vi "eDIDS-24XX-FPGA1-EPTx.vi"() -> ()   [LabVIEW 2015, in "ECS-FPGA.lvlib"]
uses:
  ECS-FPGA.lvlib
  <vilib>/Powertrain Controls/Device Drivers/Engine Position Tracking/EPTx/RevA/FPGA/Controls/EPTxTooth.ctl
  <vilib>/Powertrain Controls/Device Drivers/Engine Position Tracking/EPTx/RevA/FPGA/Controls/EPTxControl.ctl
  <vilib>/Powertrain Controls/Device Drivers/Engine Position Tracking/EPTx/RevA/FPGA/Controls/EPTxConfig.ctl
  <vilib>/Powertrain Controls/Device Drivers/Engine Position Tracking/EPTx/RevA/FPGA/Controls/EPTxSupervisor.ctl
  <vilib>/Powertrain Controls/Device Drivers/Engine Position Tracking/EPTx/RevA/FPGA/Controls/EPTxAAPControl.ctl
  <vilib>/Platform/TimedLoop/XDataNode/timing_clust.ctl
  <vilib>/Platform/TimedLoop/XDataNode/nitl_modes.ctl
  <vilib>/Platform/TimedLoop/XDataNode/wakeup.ctl
  <vilib>/Powertrain Controls/Device Drivers/Engine Position Tracking/EPTx/RevA/FPGA/Controls/EPTxSignals.ctl
  <vilib>/rvi/Emulation/niFpgaGetClockAttributes.vi
  <vilib>/rvi/Emulation/niFpgaSctlEmulationGetInTimedLoop.vi
  <vilib>/rvi/Emulation/niFpgaEmulationReportErrorSimple.vi
  <vilib>/rvi/eio/common/nirviEmuTemplateMethod_errors.vi
  <vilib>/rvi/Emulation/niFpgaCriticalErrorInLSC.vi
  <vilib>/eio/EIONode/EIONode.xnode
  <vilib>/Platform/TimedLoop/XDataNode/XDataNode.xnode
  <vilib>/Platform/TimedLoop/XDataNode/XDNodeRunTimeDep.lvlib
  <vilib>/Powertrain Controls/Device Drivers/Engine Position Tracking/EPTx/RevA/FPGA/EPTx - RevA - FPGA.lvlib
panel:
  in  "EPTx.Aux4":u8
  in  "EPTx.Aux2":u8
  in  "DI-4.PlsGen_Config_Channel3":T1
  in  "DI-4.PlsGen_Config_Channel2":T1
  in  "DI-4.PlsGen_Config_Channel1":T1
  out "DI-4.Data":T2 caption="DIData"
  out "DI-4.ScopeData":T3 caption="DIScopeData"
  in  "DI-4.ScopeRead":bool caption="DIScopeRead"
  in  "DI-4.IPhaseInterface":T4(array[cluster]) caption="IPhaseInterface"
  in  "DI-4.Control":T5 caption="DIControl"
  in  "DI-3.PlsGen_Config_Channel3":T1
  in  "DI-3.PlsGen_Config_Channel2":T1
  in  "DI-3.PlsGen_Config_Channel1":T1
  out "DI-3.Data":T2 caption="DIData"
  out "DI-3.ScopeData":T3 caption="DIScopeData"
  in  "DI-3.ScopeRead":bool caption="DIScopeRead"
  in  "DI-3.IPhaseInterface":T4(array[cluster]) caption="IPhaseInterface"
  in  "DI-3.Control":T5 caption="DIControl"
  in  "DI-2.PlsGen_Config_Channel3":T1
  in  "DI-2.PlsGen_Config_Channel2":T1
  in  "DI-2.PlsGen_Config_Channel1":T1
  out "DI-2.Data":T2 caption="DIData"
  out "DI-2.ScopeData":T3 caption="DIScopeData"
  in  "DI-2.ScopeRead":bool caption="DIScopeRead"
  in  "DI-2.IPhaseInterface":T4(array[cluster]) caption="IPhaseInterface"
  in  "DI-2.Control":T5 caption="DIControl"
  in  "DI-1.Control":T5 caption="DIControl"
  in  "DI-1.IPhaseInterface":T4(array[cluster]) caption="IPhaseInterface"
  in  "DI-1.ScopeRead":bool caption="DIScopeRead"
  out "DI-1.ScopeData":T3 caption="DIScopeData"
  out "DI-1.Data":T2 caption="DIData"
  in  "DI-1.PlsGen_Config_Channel1":T1
  in  "DI-1.PlsGen_Config_Channel2":T1
  in  "DI-1.PlsGen_Config_Channel3":T1
  in  "EPTx.Aux1AngleCapture":T6
  in  "EPTx.Aux2AngleCapture":T6
  out "EPTx.Aux1EdgeCount":u8
  out "EPTx.Aux2EdgeCount":u8
  out "EPTx.Aux1CaptureCAD":fxp<+,18,11>
  out "EPTx.Aux2CaptureCAD":fxp<+,18,11>
  in  "EPTx.Aux3AngleCapture":T6
  in  "EPTx.Aux4AngleCapture":T6
  out "EPTx.Aux3EdgeCount":u8
  out "EPTx.Aux4EdgeCount":u8
  out "EPTx.Aux3CaptureCAD":fxp<+,18,11>
  out "EPTx.Aux4CaptureCAD":fxp<+,18,11>
  in  "EPTx.Aux3":u8
  in  "EPTx.Primary":u8
  in  "EPTx.Aux1":u8
  out "EPTxSupervisor":T7
  in  "EPTxConfig":T8
  in  "EPTxControl":T9
  out "EPTxTooth":T10
  out "9411-2.DigitalTriggers":u32
  out "9220-1/AI15":fxp<+/-,24,5>
  out "9220-1/AI14":fxp<+/-,24,5>
  out "9220-1/AI13":fxp<+/-,24,5>
  out "9220-1/AI12":fxp<+/-,24,5>
  out "9220-1/AI11":fxp<+/-,24,5>
  out "9220-1/AI10":fxp<+/-,24,5>
  out "9220-1/AI9":fxp<+/-,24,5>
  out "9220-1/AI8":fxp<+/-,24,5>
  out "9220-1/AI7":fxp<+/-,24,5>
  out "9220-1/AI6":fxp<+/-,24,5>
  out "9220-1/AI5":fxp<+/-,24,5>
  out "9220-1/AI4":fxp<+/-,24,5>
  out "9220-1/AI3":fxp<+/-,24,5>
  out "9220-1/AI2":fxp<+/-,24,5>
  out "9220-1/AI1":fxp<+/-,24,5>
  out "9220-1/AI0":fxp<+/-,24,5>
  out "9411-2.5.PPWData":T11
  out "9411-2.4.PPWData":T11
  out "9411-2.3.PPWData":T11
  out "9411-2.2.PPWData":T11
  out "9411-2.1.PPWData":T11
  out "9411-2.0.PPWData":T11
  out "9411-1.5.PPWData":T11
  out "9411-1.4.PPWData":T11
  out "9411-1.3.PPWData":T11
  out "9411-1.2.PPWData":T11
  out "9411-1.1.PPWData":T11
  out "9411-1.0.PPWData":T11
  out "9411-1.DigitalTriggers":u32
  in  "9411-2.0.Filt":u16
  in  "9411-2.1.Filt":u16
  in  "9411-2.2.Filt":u16
  in  "9411-2.3.Filt":u16
  in  "9411-2.4.Filt":u16
  in  "9411-2.5.Filt":u16
  in  "9411-2.Invert":u8
  in  "9411-1.0.Filt":u16
  in  "9411-1.1.Filt":u16
  in  "9411-1.2.Filt":u16
  in  "9411-1.3.Filt":u16
  in  "9411-1.4.Filt":u16
  in  "9411-1.5.Filt":u16
  in  "9411-1.Invert":u8
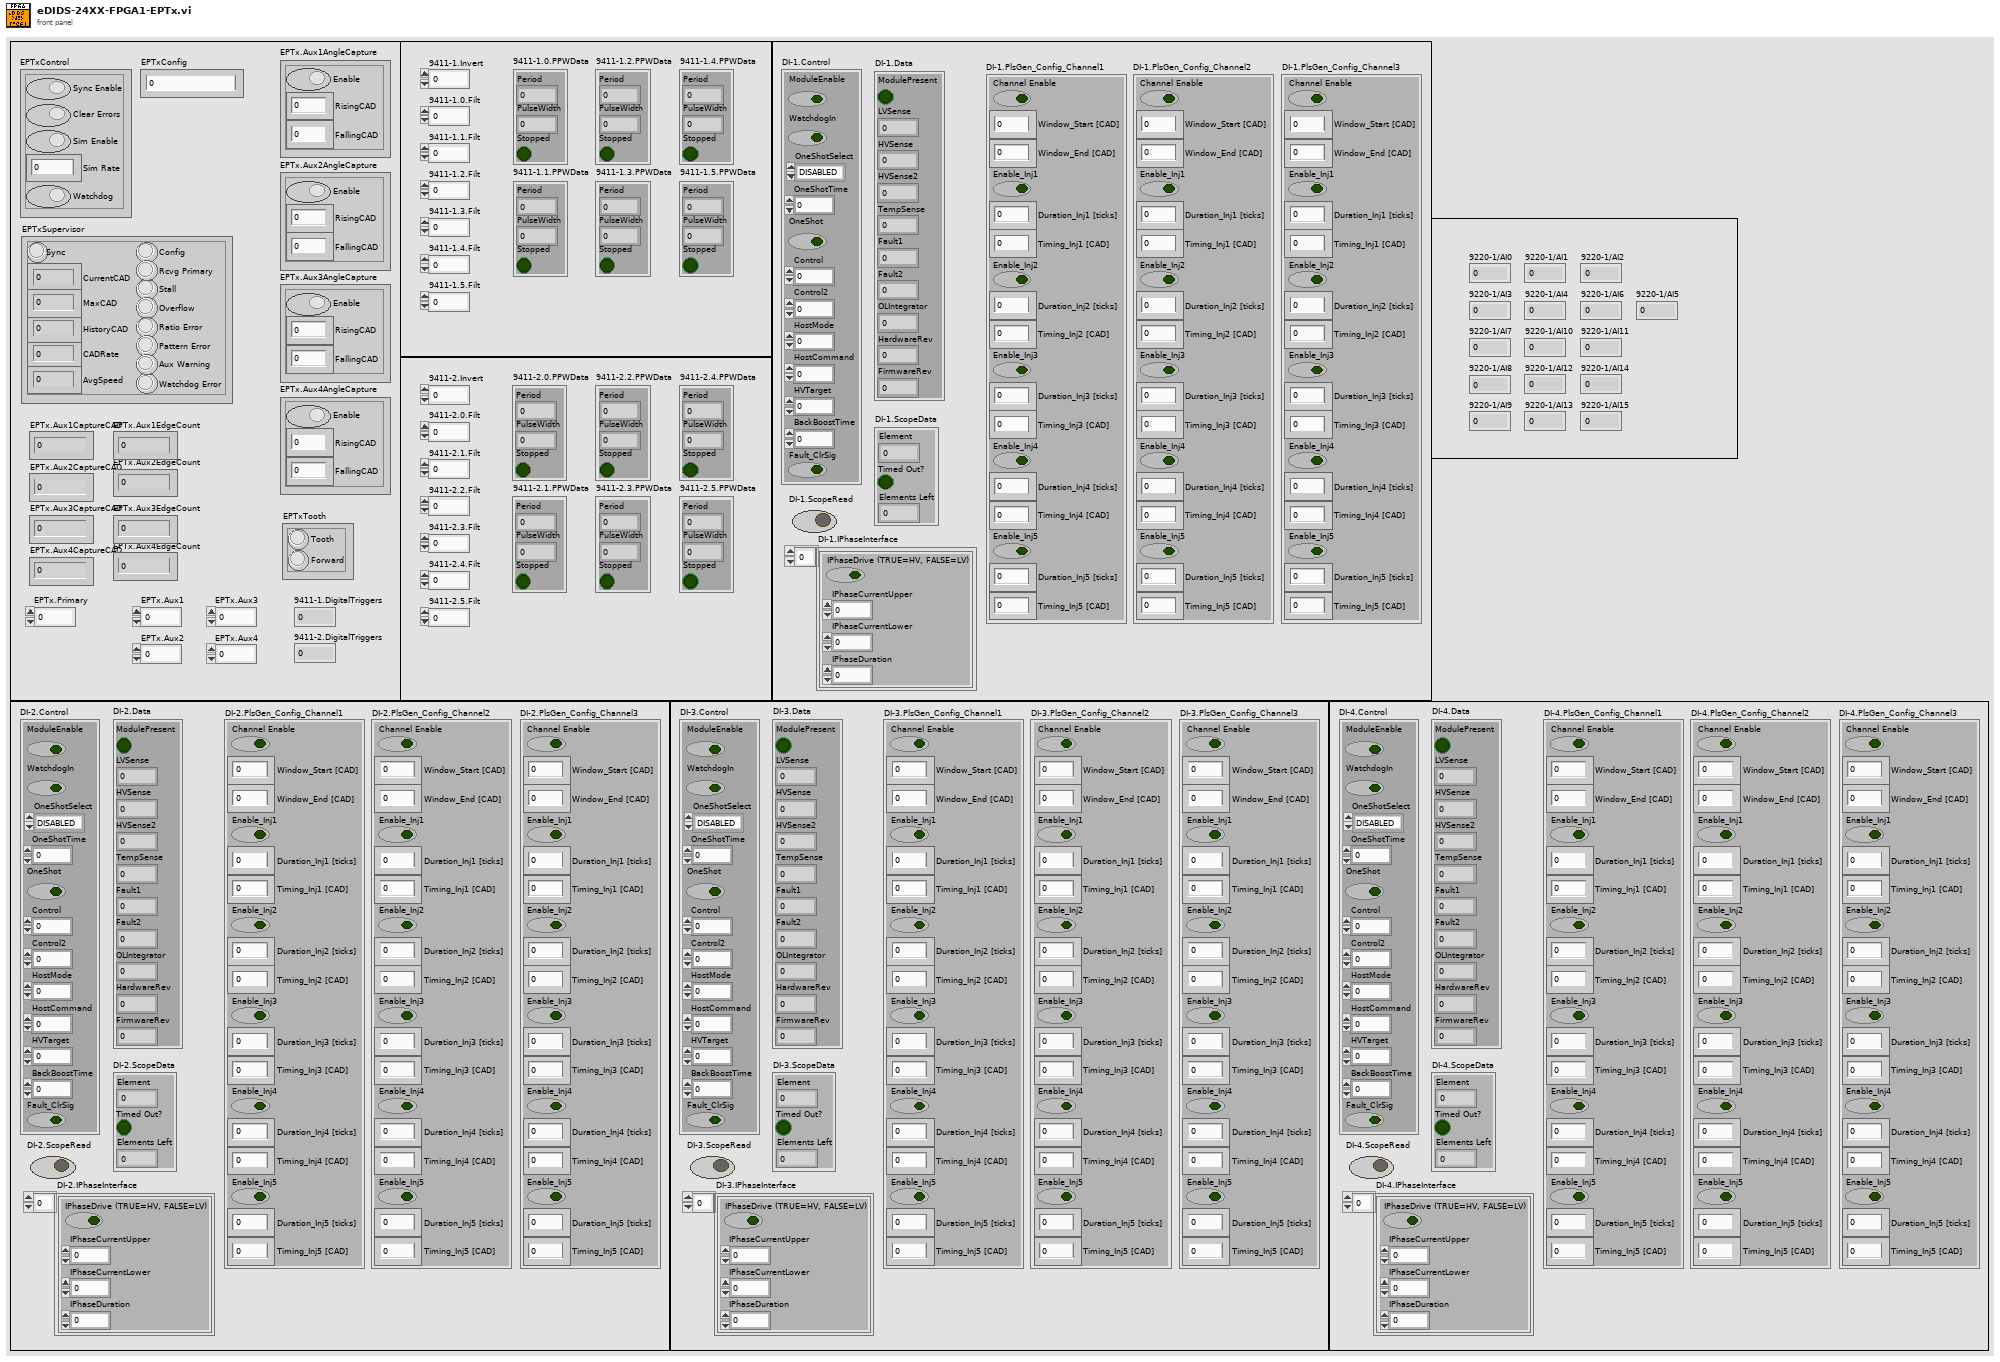
[diagram p1: front panel]
types:
  T1 = cluster{"Channel Enable":bool, "Window_Start [CAD]":fxp<+,18,11>, "Window_End [CAD]":fxp<+,18,11>, "Enable_Inj1":bool, "Duration_Inj1 [ticks]":u32, "Timing_Inj1 [CAD]":fxp<+,18,11>, "Enable_Inj2":bool, "Duration_Inj2 [ticks]":u32, "Timing_Inj2 [CAD]":fxp<+,18,11>, "Enable_Inj3":bool, "Duration_Inj3 [ticks]":u32, "Timing_Inj3 [CAD]":fxp<+,18,11>, "Enable_Inj4":bool, "Duration_Inj4 [ticks]":u32, "Timing_Inj4 [CAD]":fxp<+,18,11>, "Enable_Inj5":bool, "Duration_Inj5 [ticks]":u32, "Timing_Inj5 [CAD]":fxp<+,18,11>}
  T2 = cluster{"ModulePresent":bool, "LVSense":u8, "HVSense":u8, "HVSense2":u8, "TempSense":i8, "Fault1":u8, "Fault2":u8, "OLIntegrator":u32, "HardwareRev":u8, "FirmwareRev":u8}
  T3 = cluster{"Element":u32, "Timed Out?":bool, "Elements Left":u32}
  T4 = cluster{"IPhaseDrive (TRUE=HV, FALSE=LV)":bool, "IPhaseCurrentUpper":u16, "IPhaseCurrentLower":u16, "IPhaseDuration":u16}[]
  T5 = cluster{"ModuleEnable":bool, "WatchdogIn":bool, "OneShotSelect":enum8{"DISABLED", "CHAN 1", "CHAN 2", "CHAN 3"}, "OneShotTime":u32, "OneShot":bool, "Control":u8, "Control2":u8, "HostMode":u8, "HostCommand":u32, "HVTarget":u8, "BackBoostTime":u8, "Fault_ClrSig":bool}
  T6 = typedef "EPTx - RevA - FPGA.lvlib/EPTxAAPControl.ctl" = cluster{"Enable":bool, "RisingCAD":fxp<+,18,11>, "FallingCAD":fxp<+,18,11>}
  T7 = typedef "EPTx - RevA - FPGA.lvlib/EPTxSupervisor.ctl" = cluster{"Sync":bool, "CurrentCAD":fxp<+,18,11>, "MaxCAD":fxp<+,11,11>, "HistoryCAD":fxp<+,11,11>, "CADRate":fxp<+,22,8>, "AvgSpeed":fxp<+,17,15>, "Config":bool, "Rcvg Primary":bool, "Stall":bool, "Overflow":bool, "Ratio Error":bool, "Pattern Error":bool, "Aux Warning":bool, "Watchdog Error":bool}
  T8 = typedef "EPTx - RevA - FPGA.lvlib/EPTxConfig.ctl" = u64
  T9 = typedef "EPTx - RevA - FPGA.lvlib/EPTxControl.ctl" = cluster{"Sync Enable":bool, "Clear Errors":bool, "Sim Enable":bool, "Sim Rate":fxp<+,24,6>, "Watchdog":bool}
  T10 = typedef "EPTx - RevA - FPGA.lvlib/EPTxTooth.ctl" = cluster{"Tooth":bool, "Forward":bool}
  T11 = cluster{"Period":u32, "PulseWidth":u32, "Stopped":bool}
  T12 = typedef "XDNodeRunTimeDep.lvlib/timing_clust.ctl" = cluster{"Expected End [f-1]":u64, "Actual End [f-1]":u64, "Finished Late? [f-1]":bool, "Expected End [i-1]":u64, "Actual End [i-1]":u64, "Finished Late? [i-1]":bool, "Expected Start [i]":u64, "Actual Start [i]":u64, "Expected Start [f]":u64, "Actual Start [f]":u64, "Source Name":string, "Structure Name":string, "Period":i64, "Deadline":i64, "Offset":i64, "Start":i64, "Priority":i32, "Timeout":i32, "Mode":T13, "Wakeup Reason":T14, "Error":errorcluster, "Source Type":string, "Secondary Source Type":string, "Global End Time":u64, "Global Start Time":u64, "Frame Duration":u64, "Iteration Duration":u64, "Assigned CPU":i32, "I/O Scan Engine Mode":u32}
  T13 = typedef "XDNodeRunTimeDep.lvlib/nitl_modes.ctl" = enum32{"No Change", "Process missed periods, maintain original phase", "Discard missed periods, maintain original phase", "Process missed periods, ignore original phase", "Discard missed periods, ignore original phase"}
  T14 = typedef "XDNodeRunTimeDep.lvlib/wakeup.ctl" = enum32{"Normal", "Aborted", "Asynchronous wakeup", "Timing source error", "Timed loop error", "Timeout"}
  T15 = typedef "EPTx - RevA - FPGA.lvlib/EPTxSignals.ctl" = cluster{"Primary":bool, "Aux 1":bool, "Aux 2":bool, "Aux 3":bool, "Aux 4":bool}
  T16 = cluster{"9411-1.0.Filt":u16, "9411-1.1.Filt":u16, "9411-1.2.Filt":u16, "9411-1.3.Filt":u16, "9411-1.4.Filt":u16, "9411-1.5.Filt":u16}
  T17 = cluster{"9411-2.0.Filt":u16, "9411-2.1.Filt":u16, "9411-2.2.Filt":u16, "9411-2.3.Filt":u16, "9411-2.4.Filt":u16, "9411-2.5.Filt":u16}
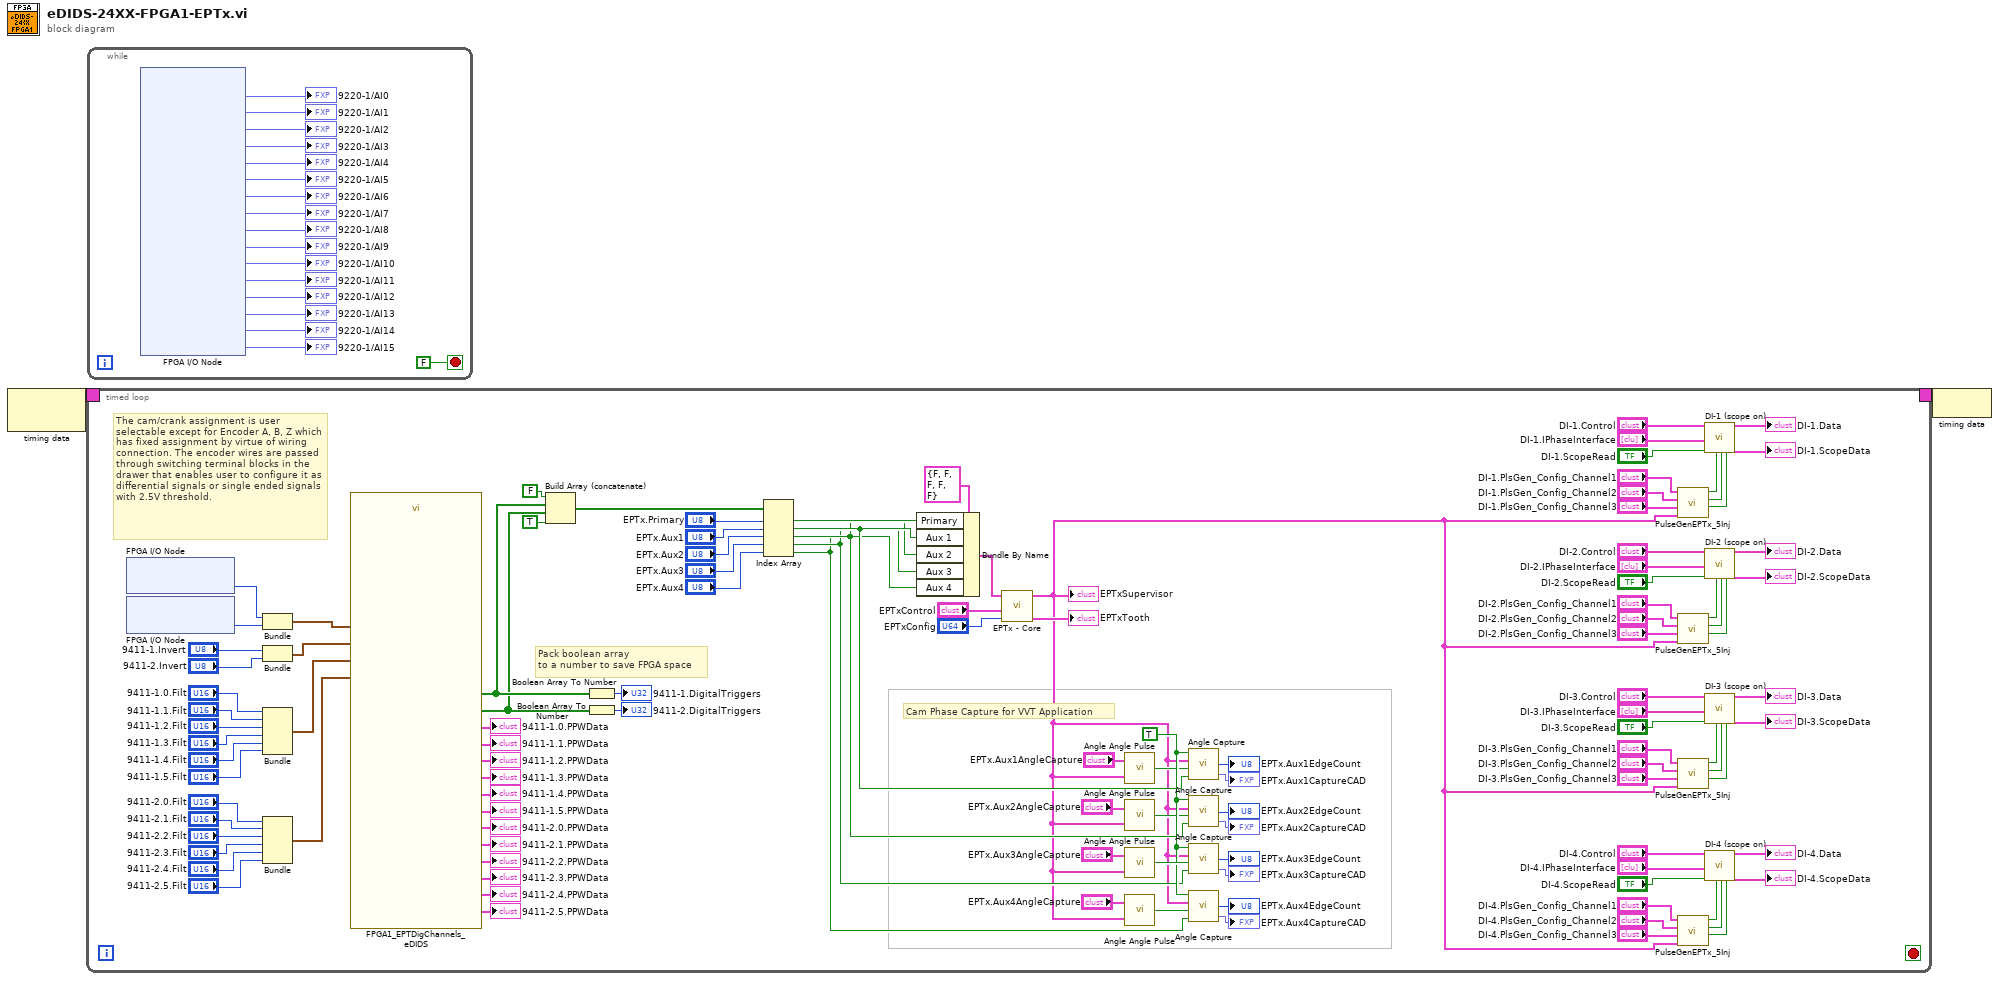
[diagram p0: block diagram]
diagram:
  n1 = node-c288() -> (w2:T12)  [unwired: 1 in]
  n2 = timed-loop {
    timing: w2 -> [_]
    timing-out: [_] -> w1
    stop <- _ stop-if-true
    w59 = TRUE ("Enable")
    # "Cam Phase Capture for VVT Application"
    # "The cam/crank assignment is user selectable except for Encoder A, B, Z which has fixed assignment by virtue of wiring connection. The encoder wires are passed through switching terminal blocks in the drawer that enables user to configure it as differential signals or single ended signals with 2.5V threshold."
    # "Pack boolean array\nto a number to save FPGA space"
    n3 = xnode "FPGA I/O Node"() -> ("9411-1/DI5:0"=w118:u8)  [unwired: 1 in, 1 out]
    n4 = xnode "FPGA I/O Node"() -> ("9411-2/DI5:0"=w117:u8)  [unwired: 1 in, 1 out]
    n5 = Bundle("9411-1/DI5:0"=w118, "9411-2/DI5:0"=w117) -> (w114:cluster{"9411-1/DI5:0":u8, "9411-2/DI5:0":u8})  [unwired: 1 in]
    n6 = Bundle("9411-1.Invert"="9411-1.Invert", "9411-2.Invert"="9411-2.Invert") -> (w113:cluster{"9411-1.Invert":u8, "9411-2.Invert":u8})  [unwired: 1 in]
    n7 = Bundle("9411-1.0.Filt"="9411-1.0.Filt", "9411-1.1.Filt"="9411-1.1.Filt", "9411-1.2.Filt"="9411-1.2.Filt", "9411-1.3.Filt"="9411-1.3.Filt", "9411-1.4.Filt"="9411-1.4.Filt", "9411-1.5.Filt"="9411-1.5.Filt") -> (w106:T16)  [unwired: 1 in]
    n8 = Bundle("9411-2.0.Filt"="9411-2.0.Filt", "9411-2.1.Filt"="9411-2.1.Filt", "9411-2.2.Filt"="9411-2.2.Filt", "9411-2.3.Filt"="9411-2.3.Filt", "9411-2.4.Filt"="9411-2.4.Filt", "9411-2.5.Filt"="9411-2.5.Filt") -> (w100:T17)  [unwired: 1 in]
    n9 = call "FPGA1_EPTDigChannels_eDIDS.vi"("9411 Inputs"=w114, "9411 Invert Commands"=w113, "9411-1.FilterValues"=w106, "9411-2.FilterValues"=w100) -> ("9411-1.0.PPWData"=→"9411-1.0.PPWData":T11, "9411-1.4.PPWData"=→"9411-1.4.PPWData":T11, "9411-1.1.PPWData"=→"9411-1.1.PPWData":T11, "9411-1.5.PPWData"=→"9411-1.5.PPWData":T11, "9411-1.2.PPWData"=→"9411-1.2.PPWData":T11, "9411-2.0.PPWData"=→"9411-2.0.PPWData":T11, "9411-1.3.PPWData"=→"9411-1.3.PPWData":T11, "9411-2.1.PPWData"=→"9411-2.1.PPWData":T11, "9411-2.2.PPWData"=→"9411-2.2.PPWData":T11, "9411-2.3.PPWData"=→"9411-2.3.PPWData":T11, "9411-2.4.PPWData"=→"9411-2.4.PPWData":T11, "9411-2.5.PPWData"=→"9411-2.5.PPWData":T11, "9411-1.DigitalTriggers"=w84:bool[], "9411-2.DigitalTriggers"=w83:bool[])  [unwired: 2 in]
    n10 = Build Array (concatenate)(FALSE, w84, w83, TRUE) -> (w72:bool[])
    n11 = Boolean Array To Number(Boolean array=w84) -> (number=→"9411-1.DigitalTriggers":u32)
    n12 = Boolean Array To Number(Boolean array=w83) -> (number=→"9411-2.DigitalTriggers":u32)
    n13 = Index Array(array=w72, index #1="EPTx.Primary", index #2="EPTx.Aux1", index #3="EPTx.Aux2", index #4="EPTx.Aux3", index #5="EPTx.Aux4") -> (element #1=w54:bool, element #2=w53:bool, element #3=w52:bool, element #4=w51:bool, element #5=w50:bool)
    n14 = Bundle By Name(cluster=T15 {"Primary"=FALSE, "Aux 1"=FALSE, "Aux 2"=FALSE, "Aux 3"=FALSE, "Aux 4"=FALSE} ("EPTxSignals"), "Primary"=w54, "Aux 1"=w53, "Aux 2"=w52, "Aux 3"=w51, "Aux 4"=w50) -> (w79:T15)
    n15 = call <vilib>:"EPTx - Core.vi"("EPTxConfig"="EPTxConfig", "EPTxControl"="EPTxControl", "EPTxSignals"=w79) -> ("EPTxTooth"=→"EPTxTooth":T10, "EPTxSupervisor"=w5:T7)  [unwired: 7 in]
    "EPTxSupervisor" <- w5
    n16 = call <vilib>:"Angle Angle Pulse.vi"("EPTxSupervisor"=w5, "AAPControl"="EPTx.Aux1AngleCapture") -> ("AAP"=w57:bool)
    n17 = call <vilib>:"Angle Angle Pulse.vi"("EPTxSupervisor"=w5, "AAPControl"="EPTx.Aux2AngleCapture") -> ("AAP"=w58:bool)
    n18 = call <vilib>:"Angle Angle Pulse.vi"("EPTxSupervisor"=w5, "AAPControl"="EPTx.Aux3AngleCapture") -> ("AAP"=w64:bool)
    n19 = call <vilib>:"Angle Angle Pulse.vi"("EPTxSupervisor"=w5, "AAPControl"="EPTx.Aux4AngleCapture") -> ("AAP"=w67:bool)
    n20 = call <vilib>:"Angle Capture.vi"("Capture"=w53, "OpWindow"=w57, "EPTxSupervisor"=w5, "Enable"=w59) -> ("CaptureCAD"=→"EPTx.Aux1CaptureCAD":fxp<+,18,11>, "CaptureCount"=→"EPTx.Aux1EdgeCount":u8)  [unwired: 1 out]
    n21 = call <vilib>:"Angle Capture.vi"("Capture"=w52, "OpWindow"=w58, "EPTxSupervisor"=w5, "Enable"=w59) -> ("CaptureCAD"=→"EPTx.Aux2CaptureCAD":fxp<+,18,11>, "CaptureCount"=→"EPTx.Aux2EdgeCount":u8)  [unwired: 1 out]
    n22 = call <vilib>:"Angle Capture.vi"("Capture"=w51, "OpWindow"=w64, "EPTxSupervisor"=w5, "Enable"=w59) -> ("CaptureCAD"=→"EPTx.Aux3CaptureCAD":fxp<+,18,11>, "CaptureCount"=→"EPTx.Aux3EdgeCount":u8)  [unwired: 1 out]
    n23 = call <vilib>:"Angle Capture.vi"("Capture"=w50, "OpWindow"=w67, "EPTxSupervisor"=w5, "Enable"=w59) -> ("CaptureCAD"=→"EPTx.Aux4CaptureCAD":fxp<+,18,11>, "CaptureCount"=→"EPTx.Aux4EdgeCount":u8)  [unwired: 1 out]
    n24 = call "PulseGenEPTx_5Inj.vi"("EPTxSupervisor"=w5, "Inj_Config_Channel3"="DI-1.PlsGen_Config_Channel3", "Inj_Config_Channel2"="DI-1.PlsGen_Config_Channel2", "Inj_Config_Channel1"="DI-1.PlsGen_Config_Channel1") -> ("CmdOut3"=w46:bool, "CmdOut2"=w45:bool, "CmdOut1"=w44:bool)  [unwired: 3 in]
    n25 = call "PulseGenEPTx_5Inj.vi"("EPTxSupervisor"=w5, "Inj_Config_Channel3"="DI-2.PlsGen_Config_Channel3", "Inj_Config_Channel2"="DI-2.PlsGen_Config_Channel2", "Inj_Config_Channel1"="DI-2.PlsGen_Config_Channel1") -> ("CmdOut3"=w31:bool, "CmdOut2"=w32:bool, "CmdOut1"=w33:bool)  [unwired: 3 in]
    n26 = call "PulseGenEPTx_5Inj.vi"("EPTxSupervisor"=w5, "Inj_Config_Channel3"="DI-3.PlsGen_Config_Channel3", "Inj_Config_Channel2"="DI-3.PlsGen_Config_Channel2", "Inj_Config_Channel1"="DI-3.PlsGen_Config_Channel1") -> ("CmdOut3"=w24:bool, "CmdOut2"=w23:bool, "CmdOut1"=w22:bool)  [unwired: 3 in]
    n27 = call "PulseGenEPTx_5Inj.vi"("EPTxSupervisor"=w5, "Inj_Config_Channel3"="DI-4.PlsGen_Config_Channel3", "Inj_Config_Channel2"="DI-4.PlsGen_Config_Channel2", "Inj_Config_Channel1"="DI-4.PlsGen_Config_Channel1") -> ("CmdOut3"=w9:bool, "CmdOut2"=w10:bool, "CmdOut1"=w11:bool)  [unwired: 3 in]
    n28 = call "DI-1 (scope on)"("DI-1_Control"="DI-1.Control", "DI-1_IPhaseInterface"="DI-1.IPhaseInterface", "DI-1_ScopeRead"="DI-1.ScopeRead", "DI1Cmd"=w44, "DI2Cmd"=w45, "DI3Cmd"=w46) -> ("DI-1_Data"=→"DI-1.Data":T2, "DI-1_ScopeData"=→"DI-1.ScopeData":T3)  [unwired: 11 in, 1 out]
    n29 = call "DI-2 (scope on)"("DI-2_Control"="DI-2.Control", "DI-2_IPhaseInterface"="DI-2.IPhaseInterface", "DI-2_ScopeRead"="DI-2.ScopeRead", "DI1Cmd"=w33, "DI2Cmd"=w32, "DI3Cmd"=w31) -> ("DI-2_Data"=→"DI-2.Data":T2, "DI-2_ScopeData"=→"DI-2.ScopeData":T3)  [unwired: 11 in, 1 out]
    n30 = call "DI-3 (scope on)"("DI-3_Control"="DI-3.Control", "DI-3_IPhaseInterface"="DI-3.IPhaseInterface", "DI-3_ScopeRead"="DI-3.ScopeRead", "DI1Cmd"=w22, "DI2Cmd"=w23, "DI3Cmd"=w24) -> ("DI-3_Data"=→"DI-3.Data":T2, "DI-3_ScopeData"=→"DI-3.ScopeData":T3)  [unwired: 11 in, 1 out]
    n31 = call "DI-4 (scope on)"("DI-4_Control"="DI-4.Control", "DI-4_IPhaseInterface"="DI-4.IPhaseInterface", "DI-4_ScopeRead"="DI-4.ScopeRead", "DI1Cmd"=w11, "DI2Cmd"=w10, "DI3Cmd"=w9) -> ("DI-4_Data"=→"DI-4.Data":T2, "DI-4_ScopeData"=→"DI-4.ScopeData":T3)  [unwired: 11 in, 1 out]
  }
  n32 = while {
    stop <- FALSE stop-if-true
    n33 = xnode "FPGA I/O Node"() -> ("9220-1/AI0"=→"9220-1/AI0":fxp<+/-,24,5>, "9220-1/AI1"=→"9220-1/AI1":fxp<+/-,24,5>, "9220-1/AI2"=→"9220-1/AI2":fxp<+/-,24,5>, "9220-1/AI3"=→"9220-1/AI3":fxp<+/-,24,5>, "9220-1/AI4"=→"9220-1/AI4":fxp<+/-,24,5>, "9220-1/AI5"=→"9220-1/AI5":fxp<+/-,24,5>, "9220-1/AI6"=→"9220-1/AI6":fxp<+/-,24,5>, "9220-1/AI7"=→"9220-1/AI7":fxp<+/-,24,5>, "9220-1/AI8"=→"9220-1/AI8":fxp<+/-,24,5>, "9220-1/AI9"=→"9220-1/AI9":fxp<+/-,24,5>, "9220-1/AI10"=→"9220-1/AI10":fxp<+/-,24,5>, "9220-1/AI11"=→"9220-1/AI11":fxp<+/-,24,5>, "9220-1/AI12"=→"9220-1/AI12":fxp<+/-,24,5>, "9220-1/AI13"=→"9220-1/AI13":fxp<+/-,24,5>, "9220-1/AI14"=→"9220-1/AI14":fxp<+/-,24,5>, "9220-1/AI15"=→"9220-1/AI15":fxp<+/-,24,5>)  [unwired: 16 in, 16 out]
  }
  n34 = node-c288(w1) -> ()
